vi "Constructor_ConsoleWriter.vi"(7 "Autoshow? (f)":bool, 8 "error in (no error)":errorcluster, 11 "max queue size (5000)":i32=5000) -> (0 "error out":errorcluster, 3 "ConsoleWriter out":refnum<class "ConsoleWriter.lvclass">)   [LabVIEW 2024, in "ConsoleWriter.lvclass"]
uses:
  ConsoleWriter.lvclass
  ConsoleWriter.lvclass/ConsoleWriter.ctl
  daemon.vi
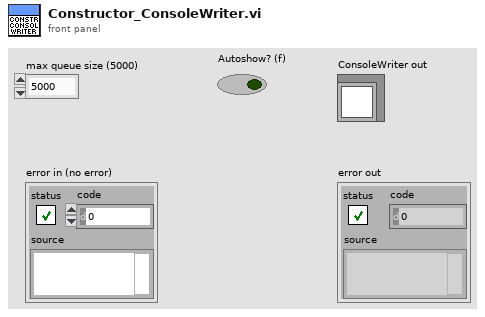
[diagram p1: front panel]
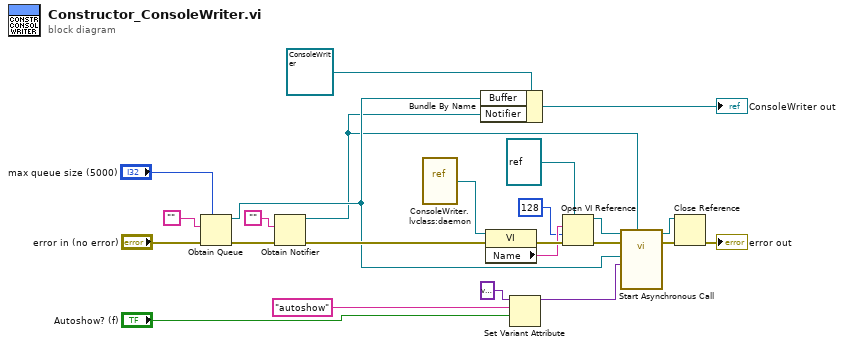
[diagram p0: block diagram]
diagram:
  n1 = Obtain Queue(max queue size (-1, unlimited)="max queue size (5000)", element data type="", error in (no error)="error in (no error)") -> (queue out=w2:refnum<queue>, error out=w3:errorcluster)  [unwired: 2 in, 1 out]
  n2 = Obtain Notifier(notification data type="", error in (no error)=w3) -> (notifier out=w1:refnum<notifier>, error out=w17:errorcluster)  [unwired: 2 in, 1 out]
  n3 = vi-ref "ConsoleWriter.lvclass:daemon.vi"() -> (w21:refnum<vi>)
  n4 = Bundle By Name(cluster=refnum<class "ConsoleWriter.lvclass"> refnum ("ConsoleWriter in"), "Buffer"=w2, "Notifier"=w1) -> (→"ConsoleWriter out":refnum<class "ConsoleWriter.lvclass">)
  n5 = property class="VI"(reference=w21, error in=w17) -> (error out=w23:errorcluster, "Name"=w22:string)  [unwired: 1 out]
  n6 = Set Variant Attribute(Variant=variant, name="autoshow", value="Autoshow? (f)") -> (Variant out=w7:variant)  [unwired: 1 in, 2 out]
  n7 = Open VI Reference(type specifier VI Refnum (for type only)=refnum<vi> refnum, vi path=w22, options=128, error in (no error)=w23) -> (vi reference=w19:refnum<vi>, error out=w20:errorcluster)  [unwired: 2 in]
  n8 = call-by-ref "Start Asynchronous Call"(reference=w19, error in=w20, "Watchdog"=w1, "args"=w7, "Buffer"=w2) -> (reference out=w12:refnum<vi>, error out=w14:errorcluster)  [unwired: 9 in]
  n9 = Close Reference(reference=w12, error in (no error)=w14) -> (error out=→"error out":errorcluster)
